vi "Array Fungsion.vi"() -> ()   [LabVIEW 2015]
panel:
  out "Index Col 5":dbl[](array[numeric])
  out "Index Row 2":dbl[](array[numeric])
  out "reversed array":dbl[](array[numeric])
  out "Index 1,4":dbl
  out "Index 3,5":dbl
  in  "2D Array":dbl[][](array[numeric])
  out "Index 3":dbl
  out "Index 0":dbl
  out "Index 7":dbl
  in  "1D Array":dbl[](array[numeric])
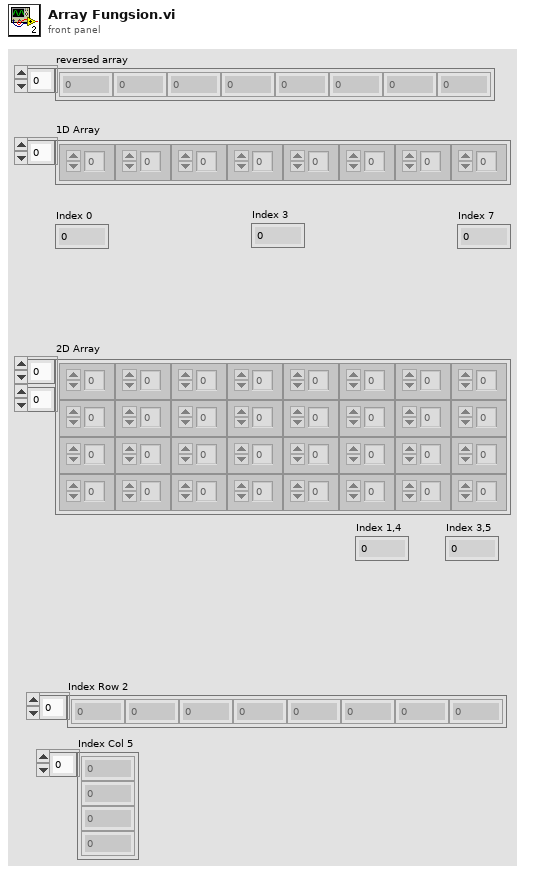
[diagram p1: front panel]
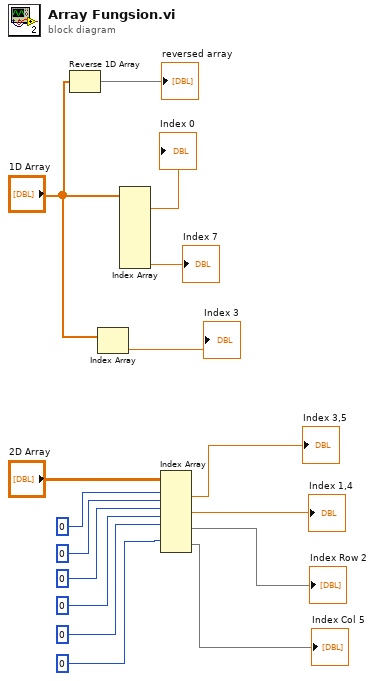
[diagram p0: block diagram]
diagram:
  n1 = Reverse 1D Array(array="1D Array") -> (reversed array=→"reversed array":dbl[])
  n2 = Index Array(array="1D Array") -> (element=→"Index 3":dbl)  [unwired: 1 in]
  n3 = Index Array "Index Array"(array="1D Array") -> (element #1=→"Index 0":dbl, element #8=→"Index 7":dbl)  [unwired: 8 in, 6 out]
  n4 = Index Array(array="2D Array", index (row) #1=0, index (col) #1=0, index (row) #2=0, index (col) #2=0, index (row) #3=0, index (row) #4=0) -> (element #1=→"Index 3,5":dbl, element #2=→"Index 1,4":dbl, element #3=→"Index Row 2":dbl[], element #4=→"Index Col 5":dbl[])  [unwired: 2 in]
